vi "Get Data Clock.vi"(0 "gen":refnum<class "niUSRP Tx DSP v2 FPGA.lvclass">) -> (4 "data clock":refnum<k21>)   [LabVIEW 2025, in "niUSRP Tx DSP v2 FPGA.lvclass"]
uses:
  niUSRP Tx DSP v2 FPGA.lvclass
  niUSRP Tx DSP v2 FPGA.lvclass/niUSRP Tx DSP v2 FPGA.ctl
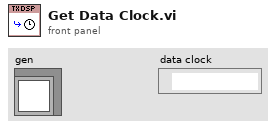
[diagram p1: front panel]
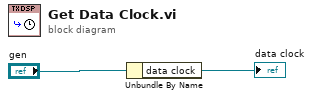
[diagram p0: block diagram]
diagram:
  n1 = Unbundle By Name("gen") -> ("data clock"=→"data clock":refnum<k21>)
